vi "FPGA.vi"() -> ()   [LabVIEW 2015]
uses:
  <vilib>/rvi/Emulation/niFpgaGetClockAttributes.vi
  <vilib>/rvi/Emulation/niFpgaSctlEmulationGetInTimedLoop.vi
  <vilib>/rvi/Emulation/niFpgaEmulationReportErrorSimple.vi
  <vilib>/rvi/eio/common/nirviEmuTemplateMethod_errors.vi
  <vilib>/rvi/interface/RandomDataEmulation/niFpgaRandomDataHandleErrors.vi
  <vilib>/rvi/Emulation/niFpgaCriticalErrorInLSC.vi
  <vilib>/rvi/FXPMathLib/FxpInterpret/XNode/nifxpmath_Interpret.xnode
  <vilib>/eio/EIONode/EIONode.xnode
  <vilib>/rvi/DataTransferAndStorage/Container/XNode/niFpgaContainer.xnode
  <vilib>/rvi/interface/RandomDataEmulation/nirviRandomDataFpgaReadWriteTemplate.vi
panel:
  in  "y":fxp<+/-,16,1>
  out "Actual Sample Rate":u32
  in  "stop":bool
  in  "frequency (periods/tick)":fxp<+,32,0>=0.0002500000409781933
  in  "Sample Rate":u32
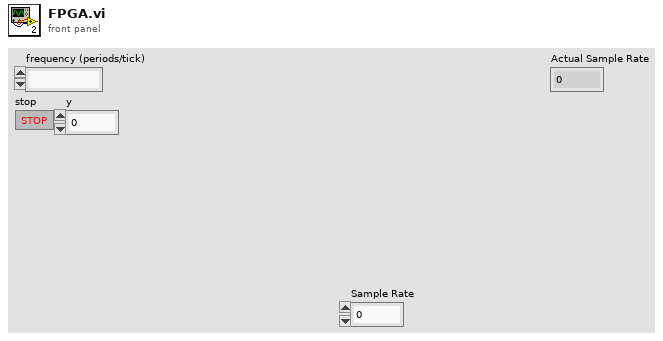
[diagram p1: front panel]
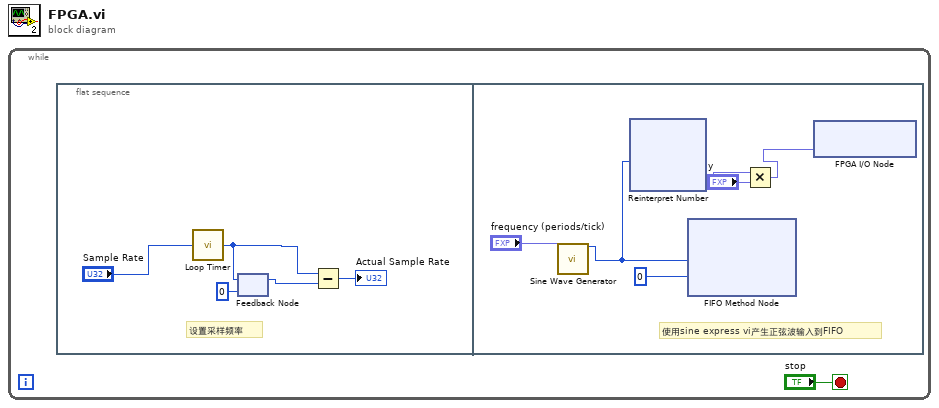
[diagram p0: block diagram]
diagram:
  n1 = while {
    stop <- "stop" stop-if-true
    n2 = flat-sequence {
      frame #0 {
        # "设置采样频率"
        n3 = call "Loop Timer"("Count(Ticks)"="Sample Rate") -> ("Tick Count(Ticks)"=w5:u32)
        n4 = feedback-in #1(w5) -> ()
        n5 = feedback #1(u32 0 ("Tick Count(Ticks)")) -> (w6:u32)
        n6 = Subtract(x=w5, y=w6) -> (x-y=→"Actual Sample Rate":u32)
      }
      frame #1 {
        # "使用sine express vi产生正弦波输入到FIFO"
        n7 = call "Sine Wave Generator"("frequency (periods/tick)"="frequency (periods/tick)") -> ("sine out"=w10:i16)  [unwired: 14 in]
        n8 = xnode "Reinterpret Number"("x"=w10) -> ("y"=w9:fxp<+/-,16,5>)
        n9 = xnode ("FIFO Method Node")("Element"=w10, "Timeout"=0) -> ()  [unwired: 1 in, 2 out]
        n10 = Multiply(x=w9, y="y") -> (x*y=w7:fxp<+/-,32,6>)
        n11 = xnode "FPGA I/O Node"("Mod2/AO0"=w7) -> ()  [unwired: 1 in, 1 out]
      }
    }
  }
